vi "Get errors.vi"(8 "error in (no error)":errorcluster, 11 "Sensor General Class in":refnum<class "Sensor General Class.lvclass">) -> (0 "error out":errorcluster, 2 "Errors":bool[](array[boolean]), 3 "Sensor General Class out":refnum<class "Sensor General Class.lvclass">)   [LabVIEW 2020, in "Sensor General Class.lvclass"]
uses:
  Sensor General Class.lvclass
  Sensor General Class.lvclass/Sensor General Class.ctl
  Data Enum.ctl
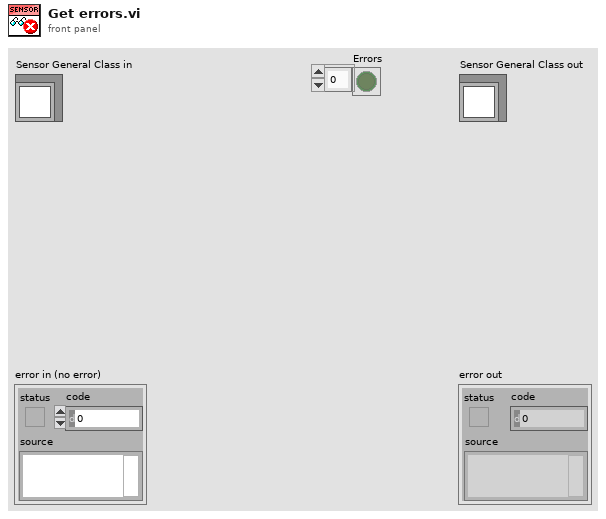
[diagram p1: front panel]
types:
  T1 = typedef "Sensor General Class.lvclass/Data Enum.ctl" = enum16{"p_bar", "p_MPa", "p_Pa", "p_kPa", "p_psi", "p_H/cm^2", "t_C", "t_K", "t_F", "rho_g/l", "rho_kg/m^3", "p20_bar", "related p20_bar", "p20_MPa", "related p20_MPa", "Tf_SF6", "Td_sf6", "tank Tf_SF6", "tank Td_SF6", "Tf_N2", "Td_N2", "tank Tf_N2", "tank Td_N2", "ppm_v SF6", "ppm_w SF6", "ppm_v N2", "ppm_w N2", "rH", "errors"}
  T2 = cluster{"Mode":enum16{"RTU", "ASCII"}, "Slave Address":u8}
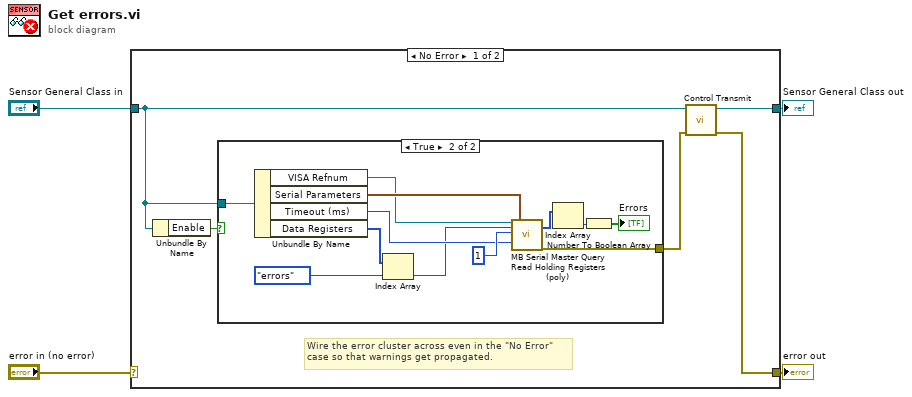
[diagram p0: block diagram]
diagram:
  n1 = case shown="No Error" "error in (no error)" {
    selector: "error in (no error)" -> [_ w23]
    tunnel: [w7 w23] -> w3
    tunnel: [w9 w22] -> w1
    tunnel: "Sensor General Class in" -> [w6 w22]
    frame No Error {
      # "Wire the error cluster across even in the \"No Error\"\ncase so that warnings get propagated."
      n2 = Unbundle By Name(w6) -> ("Enable"=w5:bool)
      n3 = case shown="True" w5 {
        tunnel: w6 -> [_ w16]
        tunnel: [_ w10] -> w8
        frame False {
        }
        frame True {
          n4 = Unbundle By Name(w16) -> ("VISA Refnum"=w20:refnum<visa-resource-name>, "Serial Parameters"=w21:T2, "Timeout (ms)"=w17:u32, "Data Registers"=w14:u16[])
          n5 = Index Array(array=w14, index=Data_Enum."errors" ("Data Enum")) -> (element=w13:u16)
          n6 = call <vilib>:"MB Serial Master Query Read Holding Registers (poly).vi"("VISA resource name"=w20, "Starting Address"=w13, "Quantity"=u16 1, "Timeout"=w17, "Serial Parameters"=w21) -> ("Holding Registers"=w19:u16[], "error out"=w10:errorcluster)  [unwired: 11 in, 2 out]
          n7 = Index Array(array=w19) -> (element=w12:u16)  [unwired: 1 in]
          n8 = Number To Boolean Array(number=w12) -> (Boolean array=→"Errors":bool[])
        }
      }
      n9 = call-dynamic "Control Transmit.vi"("error in (no error)"=w8, "Sensor General Class in"=w6) -> ("error out"=w7:errorcluster, "Sensor General Class out"=w9:refnum<class "Sensor General Class.lvclass">)  [unwired: 8 in]
    }
    frame Error {
    }
  }
  "error out" <- w3
  "Sensor General Class out" <- w1
